vi "Wait for Running.vi"(7 "Timeout (10s)":dbl=10.0, 8 "error in (no error)":errorcluster, 10 "Running":bool, 11 "Panel in":refnum<class "Panel.lvclass">) -> (0 "error out":errorcluster, 3 "Panel out":refnum<class "Panel.lvclass">)   [LabVIEW 2020, in "OOPanel.lvlib" / "Panel.lvclass"]
uses:
  <vilib>/IlluminatedG/IG OOPanel/OOPanel/Panel/Panel.lvclass
  <vilib>/IlluminatedG/IG OOPanel/OOPanel/Panel/Panel.lvclass/Panel.ctl
  <vilib>/Utility/error.llb/Error Cluster From Error Code.vi
  <vilib>/ErrorRing/Error Ring.xnode
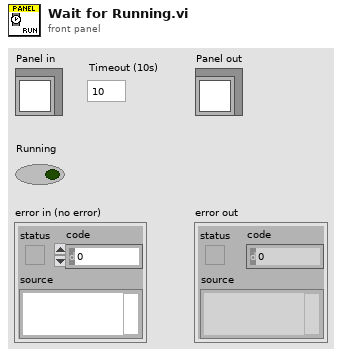
[diagram p1: front panel]
types:
  T1 = typedef "OOPanel.lvlib/Panel.lvclass/Ref Data.ctl" = cluster{"Panel Ref":refnum<vi>, "SubPanel":refnum<vi>, "Close":bool, "Running":bool, "State":T2}
  T2 = typedef "OOPanel.lvlib/Panel.lvclass/Visibility State.ctl" = enum16{"Idle", "Closed", "Hidden", "Visible", "Subpanel"}
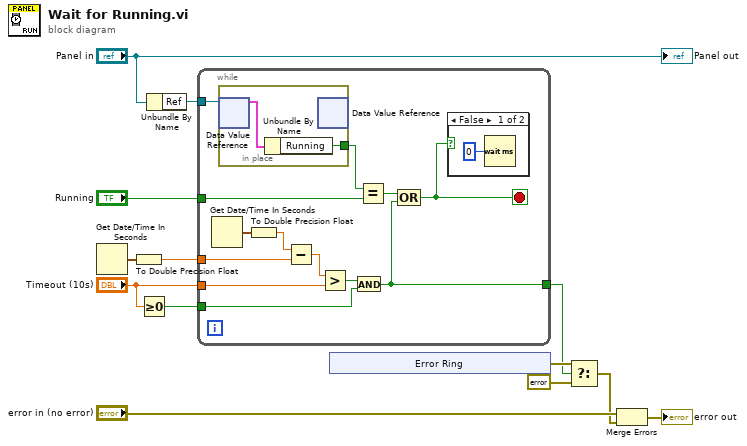
[diagram p0: block diagram]
diagram:
  n1 = Get Date/Time In Seconds() -> (seconds since 1Jan1904=w12:timestamp)
  n2 = To Double Precision Float(number=w12) -> (double precision float=w9:dbl)
  n3 = Greater Or Equal To 0?(x="Timeout (10s)") -> (x >= 0?=w6:bool)
  n4 = Unbundle By Name("Panel in") -> ("Ref"=w11:refnum<data-value>)
  n5 = while {
    tunnel: w11 -> [w26]
    tunnel: w9 -> [w24]
    tunnel: "Running" -> [w20]
    tunnel: "Timeout (10s)" -> [w22]
    tunnel: w6 -> [w16]
    tunnel: [w15] -> w4
    stop <- w14 stop-if-true
    n6 = Get Date/Time In Seconds() -> (seconds since 1Jan1904=w25:timestamp)
    n7 = in-place {
      in-place-border: [w28] -> w19
      n8 = in-place-dvr #1(w26) -> (w29:T1)  [unwired: 1 out]
      n9 = Unbundle By Name(w29) -> ("Running"=w28:bool)
      n10 = in-place-dvr #1() -> ()  [unwired: 1 in, 2 out]
    }
    n11 = To Double Precision Float(number=w25) -> (double precision float=w23:dbl)
    n12 = Subtract(x=w23, y=w24) -> (x-y=w21:dbl)
    n13 = Greater?(x=w21, y=w22) -> (0:w17:bool)
    n14 = And(x=w17, y=w16) -> (x .and. y?=w15:bool)
    n15 = Equal?(x=w19, y=w20) -> (x = y?=w18:bool)
    n16 = Compound Arithmetic op=OR(w18, w15) -> (w14:bool)
    n17 = case shown="False" w14 {
      frame False {
        n18 = Wait (ms)(milliseconds to wait=u32 0) -> ()  [unwired: 1 out]
      }
      frame True {
      }
    }
  }
  n19 = xnode "Error Ring"() -> ("error out"=w5:errorcluster)
  n20 = Select(t=w5, s=w4, f=errorcluster {"status"=FALSE, "code"=0, "source"=""}) -> (s? t:f=w1:errorcluster)
  n21 = Merge Errors("error in (no error)", w1) -> (→"error out":errorcluster)
  "Panel out" <- "Panel in"
